vi "RichToFlatsift_proxy_v1_PingResponse.vi"(5 "OutputClusterType":T1, 11 "InputCluster":T2) -> (3 "OutputCluster":T1)   [LabVIEW 2024, in "SiftProxy_client.lvlib"]
uses:
  sift_proxy_v1_PingResponse.ctl
  sift_proxy_v1_PingResponse_Flat.ctl
  SiftProxy_client.lvlib
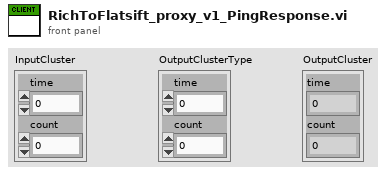
[diagram p1: front panel]
types:
  T1 = typedef "SiftProxy_client.lvlib/sift_proxy_v1_PingResponse_Flat.ctl" = cluster{"time":i64, "count":i64}
  T2 = typedef "SiftProxy_client.lvlib/sift_proxy_v1_PingResponse.ctl" = cluster{"time":i64, "count":i64}
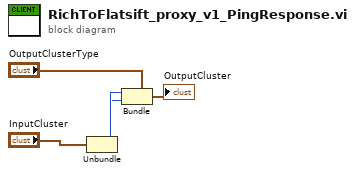
[diagram p0: block diagram]
diagram:
  n1 = Unbundle "Unbundle"("InputCluster") -> ("time"=w2:i64, "count"=w1:i64)
  n2 = Bundle "Bundle"(cluster="OutputClusterType", "time"=w2, "count"=w1) -> (→"OutputCluster":T1)
